vi "Remove State Connection.vi"(8 "error in":errorcluster, 9 "connection":T1, 10 "state":string, 11 "routing channel in":T2 format="%.0x") -> (0 "error out":errorcluster, 3 "routing channel out":T2=18446744073709551615 format="%.0x")   [LabVIEW 2020, in "Routing and Faulting Scripting.lvlib"]
doc: "Removes the connection from the state."
uses:
  Routing and Faulting Scripting.lvlib
  <vilib>/NI VeriStand/Custom Device API/Custom Device Item Ref.ctl
  Shared/Connection.ctl
  NationalInstruments.VeriStand.SystemDefinitionAPI
  Constants/Scripting Constants.vi
  <vilib>/Utility/error.llb/Error Cluster From Error Code.vi
  <vilib>/NI VeriStand/Custom Device API/Custom Device API.lvlib
  Shared/Routing and Faulting Shared.lvlib
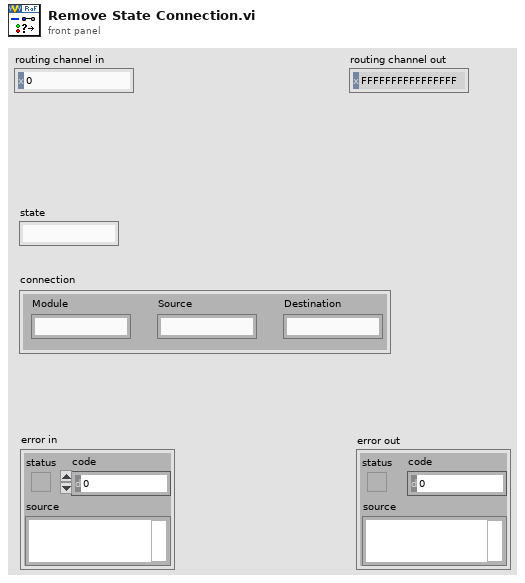
[diagram p1: front panel]
types:
  T1 = typedef "Routing and Faulting Shared.lvlib/Connection.ctl" = cluster{"Module":string, "Source":string, "Destination":string}
  T2 = typedef "Custom Device API.lvlib/Custom Device Item Ref.ctl" = u64
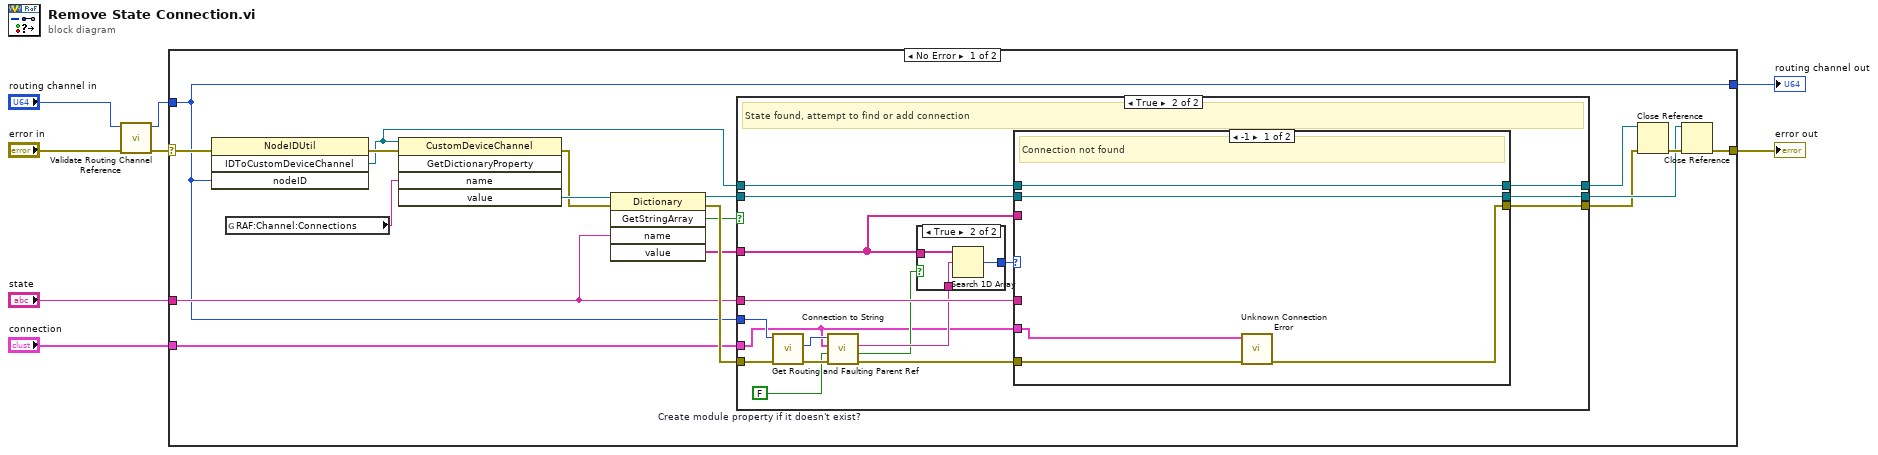
[diagram p0: block diagram]
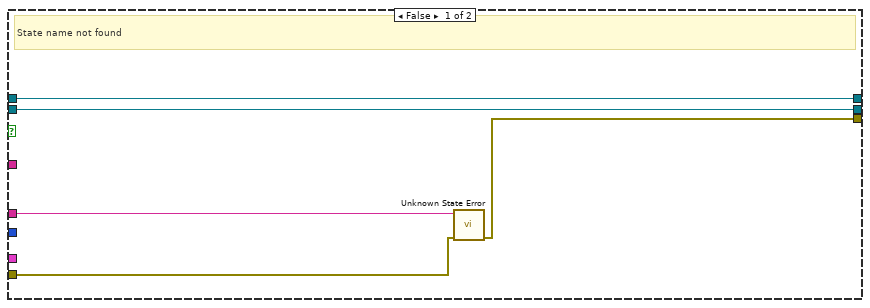
[diagram p2: hidden frame]
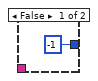
[diagram p3: hidden frame]
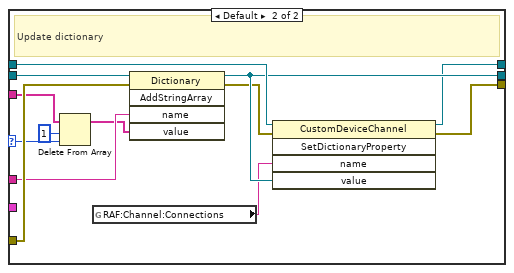
[diagram p4: hidden frame]
diagram:
  n1 = call "Validate Routing Channel Reference.vi"("error in"="error in", "routing channel in"="routing channel in") -> ("error out"=w3:errorcluster, "routing channel out"=w1:T2)  [unwired: 8 in]
  n2 = case shown="No Error" w3 {
    selector: w3 -> [w22 w72]
    tunnel: [w25 w72] -> w7
    tunnel: w1 -> [w9 w71]
    tunnel: [w9 w71] -> w6
    tunnel: "state" -> [w16 _]
    tunnel: "connection" -> [w11 _]
    frame No Error {
      n3 = invoke class="NodeIDUtil" method="IDToCustomDeviceChannel"(error in=w22, "nodeID"=w9) -> (error out=w23:errorcluster, "IDToCustomDeviceChannel"=w13:refnum<k24>)  [unwired: 2 in, 2 out]
      n4 = global read "Scripting Constants.vi" "RAF:Channel:Connections"() -> (w10:string)
      n5 = invoke class="CustomDeviceChannel" method="GetDictionaryProperty"(reference=w13, error in=w23, "name"=w10) -> (error out=w19:errorcluster, "value"=w20:refnum<k24>)  [unwired: 2 in, 3 out]
      n6 = invoke class="Dictionary" method="GetStringArray"(reference=w20, error in=w19, "name"=w16) -> (reference out=w17:refnum<k24>, error out=w26:errorcluster, "GetStringArray"=w18:bool, "value"=w21:string[])  [unwired: 2 in, 1 out]
      n7 = case shown="True" w18 {
        tunnel: w21 -> [_ w41]
        tunnel: w26 -> [w28 w38]
        tunnel: [w29 w47] -> w14
        tunnel: w16 -> [w27 w46]
        tunnel: w17 -> [w31 w45]
        tunnel: [w31 w44] -> w15
        tunnel: w13 -> [w30 w43]
        tunnel: [w30 w42] -> w12
        tunnel: w11 -> [_ w32]
        tunnel: w9 -> [_ w35]
        frame False {
          # "State name not found"
          n8 = call "Unknown State Error.vi"("error in (no error)"=w28, "state"=w27) -> ("error out"=w29:errorcluster)  [unwired: 9 in]
        }
        frame True {
          w34 = FALSE  # Create module property if it doesn't exist?
          # "State found, attempt to find or add connection"
          n9 = call "Get Routing and Faulting Parent Ref.vi"("error in"=w38, "routing and faulting child in"=w35) -> ("error out"=w37:errorcluster, "routing and faulting"=w36:T2)  [unwired: 7 in, 1 out]
          n10 = call "Connection to String.vi"("error in"=w37, "create module property if it doesn't exist? (T)"=w34, "connection"=w32, "routing and faulting in"=w36) -> ("error out"=w39:errorcluster, "conversion successful?"=w33:bool, "string"=w40:string)  [unwired: 4 in, 1 out]
          n11 = case shown="True" w33 {
            tunnel: [-1 ("index of element") w52] -> w48
            tunnel: w41 -> [_ w51]
            tunnel: w40 -> [_ w50]
            frame False {
            }
            frame True {
              n12 = Search 1D Array(1D array=w51, element=w50) -> (index of element=w52:i32)  [unwired: 1 in]
            }
          }
          n13 = case shown="-1" w48 {
            selector: w48 -> [_ w61]
            tunnel: w39 -> [w55 w70]
            tunnel: [w54 w64] -> w47
            tunnel: w46 -> [_ w69]
            tunnel: w45 -> [w57 w68]
            tunnel: [w57 w66] -> w44
            tunnel: w43 -> [w56 w67]
            tunnel: [w56 w63] -> w42
            tunnel: w41 -> [_ w62]
            tunnel: w32 -> [w53 _]
            frame -1 {
              # "Connection not found"
              n14 = call "Unknown Connection Error.vi"("error in (no error)"=w55, "connection"=w53) -> ("error out"=w54:errorcluster)  [unwired: 9 in]
            }
            frame Default {
              # "Update dictionary"
              n15 = Delete From Array(array=w62, length=1, index=w61) -> (array with subset deleted=w60:string[])  [unwired: 1 out]
              n16 = global read "Scripting Constants.vi" "RAF:Channel:Connections"() -> (w58:string)
              n17 = invoke class="Dictionary" method="AddStringArray"(reference=w68, error in=w70, "name"=w69, "value"=w60) -> (reference out=w66:refnum<k24>, error out=w65:errorcluster)  [unwired: 1 in, 3 out]
              n18 = invoke class="CustomDeviceChannel" method="SetDictionaryProperty"(reference=w67, error in=w65, "name"=w58, "value"=w66) -> (reference out=w63:refnum<k24>, error out=w64:errorcluster)  [unwired: 1 in, 3 out]
            }
          }
        }
      }
      n19 = Close Reference(reference=w12, error in (no error)=w14) -> (error out=w24:errorcluster)
      n20 = Close Reference(reference=w15, error in (no error)=w24) -> (error out=w25:errorcluster)
    }
    frame Error {
    }
  }
  "routing channel out" <- w6
  "error out" <- w7
